vi "chr63204A_CC_L1_set.vi"(8 "error in (no error)":errorcluster, 10 "CC current":dbl, 11 "VISA resource name":refnum<visa-resource-name>) -> (0 "error out":errorcluster, 3 "VISA resource name out":refnum<visa-resource-name>)   [LabVIEW 2020]
doc: "Sets the current to be loaded on chroma 63204A"
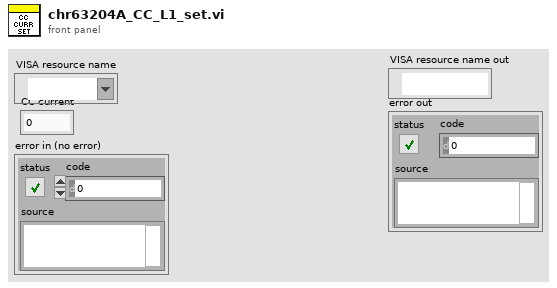
[diagram p1: front panel]
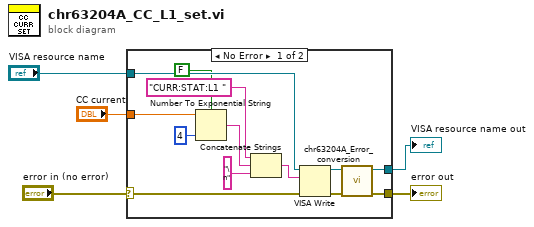
[diagram p0: block diagram]
diagram:
  n1 = case shown="No Error" "error in (no error)" {
    selector: "error in (no error)" -> [w12 w19]
    tunnel: "CC current" -> [w18 _]
    tunnel: "VISA resource name" -> [w13 w20]
    tunnel: [w11 w20] -> w2
    tunnel: [w10 w19] -> w1
    frame No Error {
      n2 = Number To Exponential String(number=w18, precision (6)=i16 4, 1:FALSE ("use system decimal point (T)")) -> (E-format string=w17:string)  [unwired: 1 in]
      n3 = Concatenate Strings("CURR:STAT:L1 " ("string"), w17, "\n" ("string")) -> (w15:string)
      n4 = VISA Write(VISA resource name=w13, write buffer=w15, error in (no error)=w12) -> (VISA resource name out=w9:refnum<visa-resource-name>, error out=w8:errorcluster)  [unwired: 1 out]
      n5 = call "chr63204A_Error_conversion.vi"("error in (no error)"=w8, "VISA resource name"=w9) -> ("error out"=w10:errorcluster, "VISA resource name out"=w11:refnum<visa-resource-name>)  [unwired: 8 in]
    }
    frame Error {
    }
  }
  "VISA resource name out" <- w2
  "error out" <- w1
